vi "Get Local Framework Path.vi"(8 "error in":errorcluster) -> (0 "error out":errorcluster, 3 "path out":path)   [LabVIEW 2019]
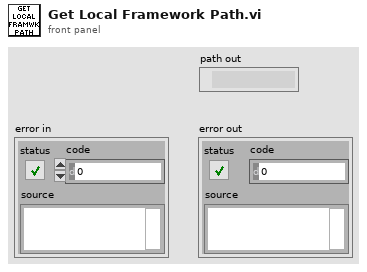
[diagram p1: front panel]
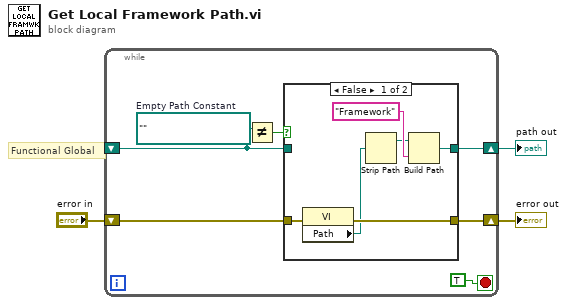
[diagram p0: block diagram]
diagram:
  # "Functional Global"
  n1 = while {
    shift-right: [w8] -> w1
    shift-left: _ -> [w4]
    shift-right: [w10] -> w3
    shift-left: "error in" -> [w9]
    stop <- TRUE stop-if-true
    w7 = path ""  # Empty Path Constant
    n2 = Not Equal?(x=w4, y=w7) -> (x != y?=w5:bool)
    n3 = case shown="False" w5 {
      tunnel: [w16 w18] -> w10
      tunnel: w9 -> [w15 w18]
      tunnel: [w14 w17] -> w8
      tunnel: w4 -> [_ w17]
      frame False {
        n4 = property class="VI"(error in=w15) -> (error out=w16:errorcluster, "Path"=w13:path)  [unwired: 1 in, 1 out]
        n5 = Strip Path(path=w13) -> (stripped path=w11:path)  [unwired: 1 out]
        n6 = Build Path(base path=w11, name or relative path="Framework") -> (appended path=w14:path)
      }
      frame True {
      }
    }
  }
  "path out" <- w1
  "error out" <- w3
